vi "read position.vi"(8 "error in (no error)":errorcluster, 11 "CL57RS in":refnum<class "CL57RS.lvclass">) -> (0 "error out":errorcluster, 2 "Angle":dbl, 3 "CL57RS out":refnum<class "CL57RS.lvclass">)   [LabVIEW 2025, in "Motor.lvlib" / "CL57RS.lvclass"]
uses:
  CL57RS.lvclass
  CL57RS.lvclass/CL57RS.ctl
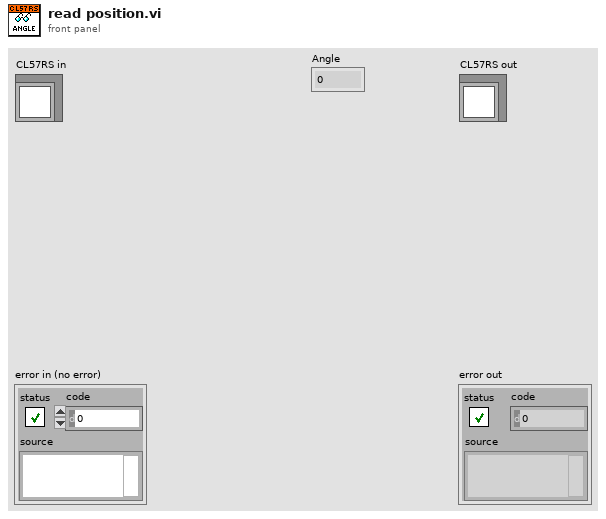
[diagram p1: front panel]
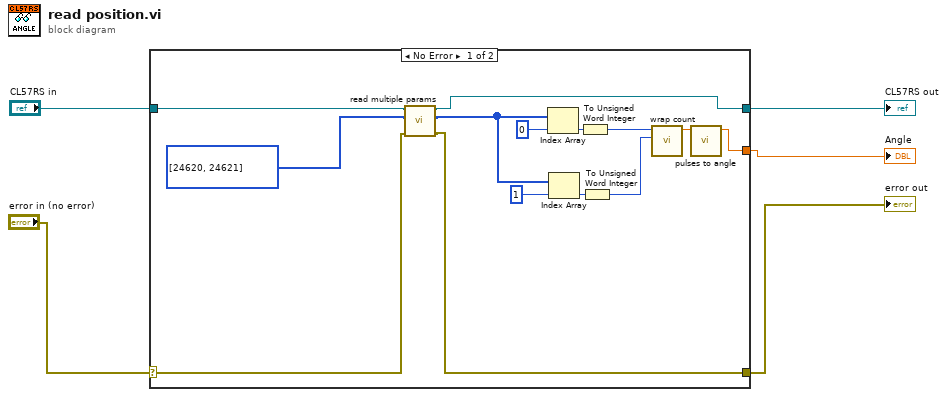
[diagram p0: block diagram]
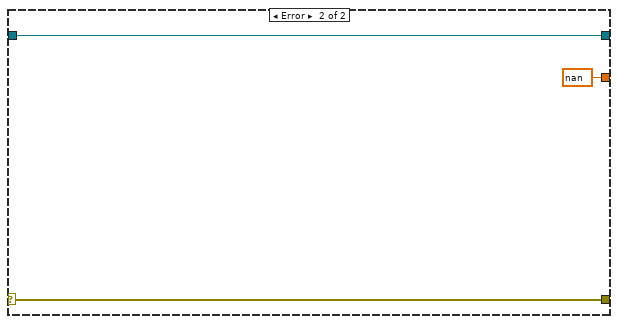
[diagram p2: hidden frame]
diagram:
  n1 = case shown="No Error" "error in (no error)" {
    selector: "error in (no error)" -> [w14 w22]
    tunnel: [w15 w22] -> w2
    tunnel: [w11 w21] -> w4
    tunnel: "CL57RS in" -> [w10 w21]
    tunnel: [w6 nan ("Angle")] -> w1
    frame No Error {
      n2 = call "read multiple params.vi"("error in (no error)"=w14, "Parameters"=u32[] [24620, 24621], "CL57RS in"=w10) -> ("error out"=w15:errorcluster, "Hex Result"=w12:u32[], "CL57RS out"=w11:refnum<class "CL57RS.lvclass">)  [unwired: 6 in]
      n3 = Index Array(array=w12, index=0) -> (element=w16:u32)
      n4 = Index Array(array=w12, index=1) -> (element=w17:u32)
      n5 = To Unsigned Word Integer(number=w16) -> (unsigned 16bit integer=w9:u16)
      n6 = To Unsigned Word Integer(number=w17) -> (unsigned 16bit integer=w8:u16)
      n7 = call "wrap count.vi"("lo"=w8, "hi"=w9) -> ("Numeric"=w7:dbl)  [unwired: 9 in]
      n8 = call "pulses to angle.vi"("Pulses"=w7) -> ("Angle"=w6:dbl)  [unwired: 10 in]
    }
    frame Error {
    }
  }
  "error out" <- w2
  "CL57RS out" <- w4
  "Angle" <- w1
